vi "Controller - State Process.vi"(8 "error in (no error)":errorcluster, 11 "View Model":T1) -> (0 "error out":errorcluster, 3 "View Model":T1)   [LabVIEW 2017]
doc: "Process state during car wash execution."
uses:
  View Model/Controls/View Model.ctl
  View Model/Controls/Shared Model.ctl
  Error Handler/Controls/Error Model.ctl
  Error Handler/Controls/Error Data.ctl
  Error Handler/Controls/Error Level.ctl
  Configuration/Controls/Config Model.ctl
  Configuration/Controls/Config Record.ctl
  Configuration/Controls/Config Data.ctl
  Configuration/Controls/Config Command.ctl
  Controls/Controler Model.ctl
  Views/Entry Console View/Controls/Entry Console - Wash Steps.ctl
  Controls/Controller - Event.ctl
  Controls/Controller - Commands.ctl
  Controls/Controller - Overhead.ctl
  Controls/Controller - States.ctl
  Controls/Controller - Wash Step.ctl
  Views/Vehicle Position View/Controls/Vehicle - Station Enum.ctl
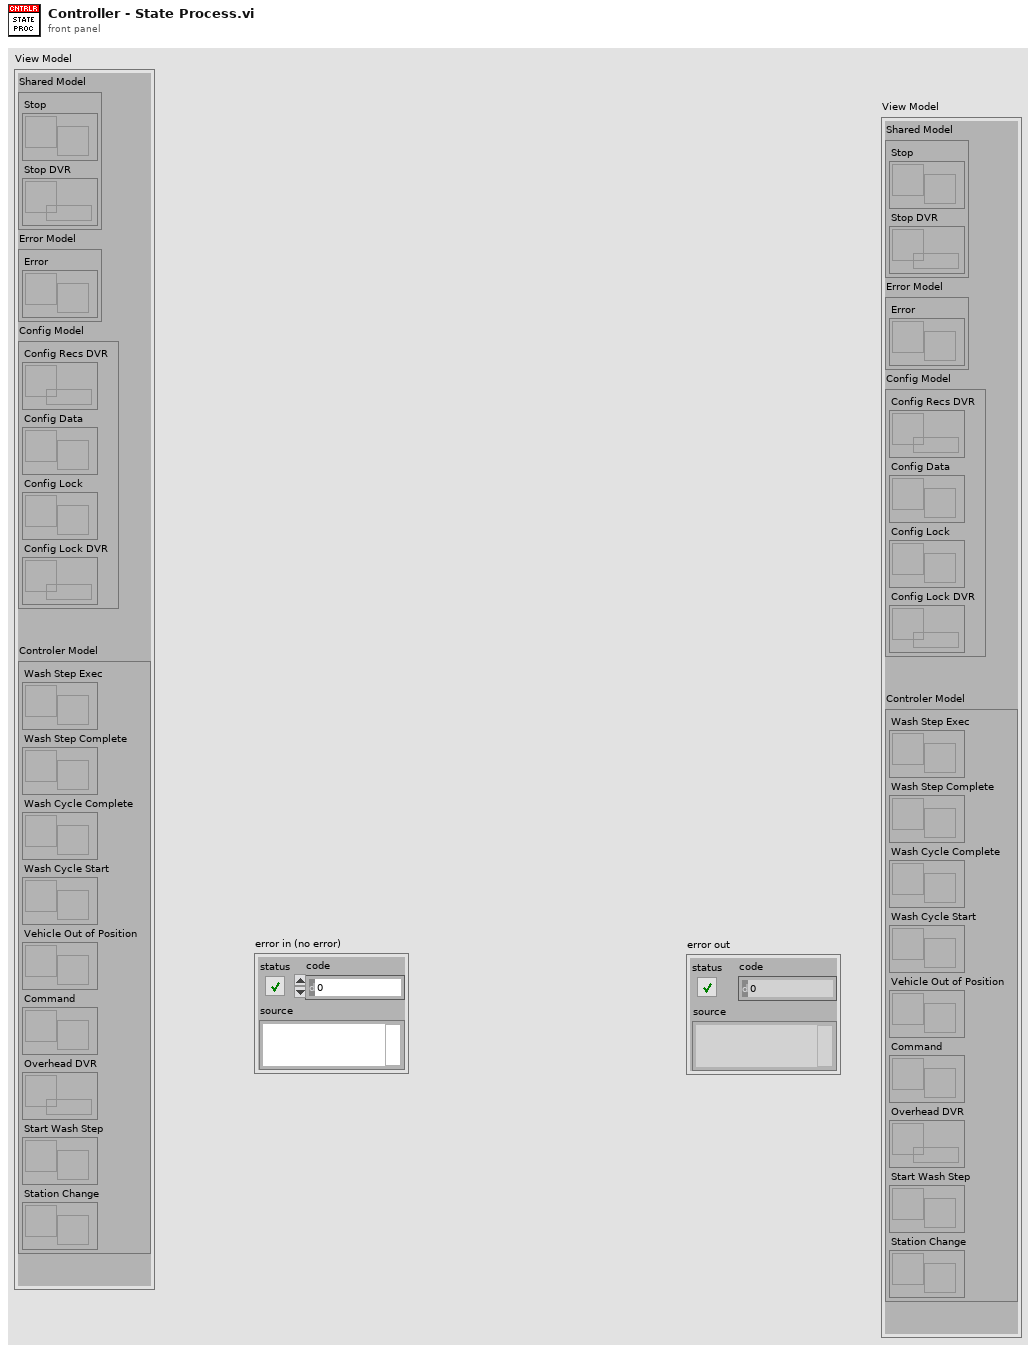
[diagram p1: front panel]
types:
  T1 = typedef "View Model.ctl" = cluster{"Shared Model":T2, "Error Model":T3, "Config Model":T4, "Controler Model":T5}
  T2 = typedef "Shared Model.ctl" = cluster{"Stop":refnum<user-event>, "Stop DVR":refnum<data-value>}
  T3 = typedef "Error Model.ctl" = cluster{"Error":refnum<user-event>}
  T4 = typedef "Config Model.ctl" = cluster{"Config Recs DVR":refnum<data-value>, "Config Data":refnum<user-event>, "Config Lock":refnum<user-event>, "Config Lock DVR":refnum<data-value>}
  T5 = typedef "Controler Model.ctl" = cluster{"Wash Step Exec":refnum<user-event>, "Wash Step Complete":refnum<user-event>, "Wash Cycle Complete":refnum<user-event>, "Wash Cycle Start":refnum<user-event>, "Vehicle Out of Position":refnum<user-event>, "Command":refnum<user-event>, "Overhead DVR":refnum<data-value>, "Start Wash Step":refnum<user-event>, "Station Change":refnum<user-event>}
  T6 = typedef "Controller - States.ctl" = enum16{"Initial", "Wait for Start", "Wash Cycle Start", "Wait for Vehicle Position", "Wash Step Start", "Wash Step Execute", "Wash Step Complete", "Wash Cycle Complete", "Wash Exit", "Wash Abort/Terminate"}
  T7 = typedef "Controller - Wash Step.ctl" = enum16{"Under Body Wash", "Bug Remover", "Pre-Soak", "High Pressure Wash", "Low Pressure Wax", "Spot Free Rinse", "Tire Shine Foam", "Air Dry"}
  T8 = typedef "Config Record.ctl" = cluster{"Wash Step":string, "Station":string, "Step Duration":u32}
  T9 = typedef "Vehicle - Station Enum.ctl" = enum16{"Entry", "Station1", "Station2", "Station3", "Exit"}
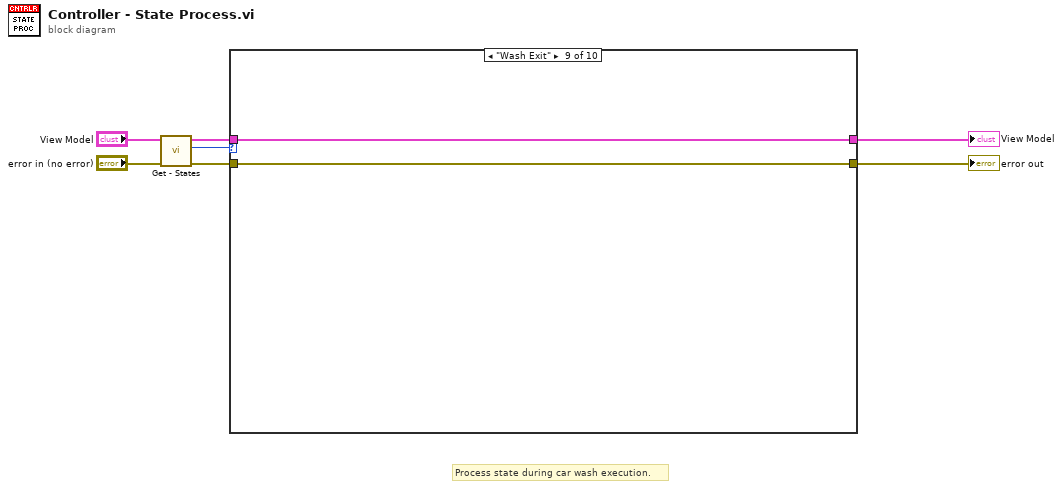
[diagram p0: block diagram]
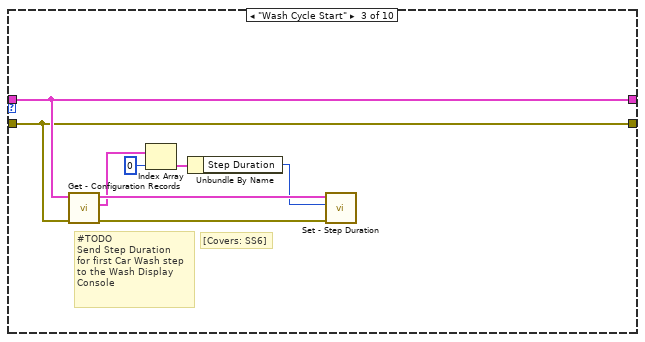
[diagram p4: hidden frame]
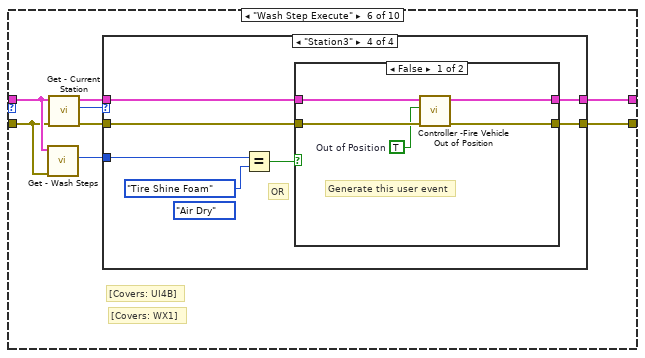
[diagram p7: hidden frame]
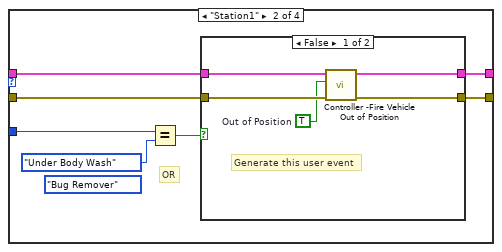
[diagram p9: hidden frame]
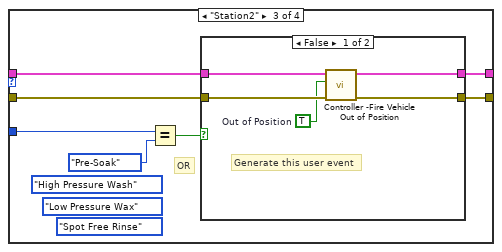
[diagram p11: hidden frame]
diagram:
  # "Process state during car wash execution."
  n1 = call "Get - States.vi"("error in (no error)"="error in (no error)", "View Model"="View Model") -> ("error out"=w3:errorcluster, "Current State"=w5:T6, "View Model"=w4:T1)  [unwired: 6 in, 1 out]
  n2 = case shown="\"Wash Exit\"" w5 {
    tunnel: w4 -> [w9 w11 w17 w21 w23 w28 w77 w79 w81 w83]
    tunnel: w3 -> [w8 w10 w16 w20 w22 w27 w76 w78 w80 w82]
    tunnel: [w9 w11 w17 w21 w23 w25 w77 w79 w81 w83] -> w1
    tunnel: [w8 w10 w16 w20 w22 w24 w76 w78 w80 w82] -> w2
    frame "Initial" {
    }
    frame "Wait for Start", Default {
      # "[Covers: WS1]"
      # "#TODO\n- Continue maintain Initial state requirements"
    }
    frame "Wash Cycle Start" {
      # "[Covers: SS6]"
      # "#TODO\nSend Step Duration\nfor first Car Wash step\nto the Wash Display \nConsole"
      n3 = call "Get - Configuration Records.vi"("error in (no error)"=w16, "View Model"=w17) -> ("error out"=w12:errorcluster, "Config Records"=w15:T8[], "View Model"=w18:T1)  [unwired: 7 in]
      n4 = Index Array(array=w15, index=0) -> (element=w14:T8)
      n5 = Unbundle By Name(w14) -> ("Step Duration"=w13:u32)
      n6 = call "Set - Step Duration.vi"("error in (no error)"=w12, "Step Duration"=w13, "View Model"=w18) -> ()  [unwired: 7 in, 2 out]
    }
    frame "Wait for Vehicle Position" {
      # "[Covers: VS4]"
      # "#TODO\nWait for user event Station\nChange to the correct station\nor to the Exit"
    }
    frame "Wash Step Start" {
    }
    frame "Wash Step Execute" {
      # "[Covers: WX1]"
      # "[Covers: UI4B]"
      n7 = call "Get - Wash Steps.vi"("error in (no error)"=w27, "View Model"=w28) -> ("Current Wash Step"=w26:T7)  [unwired: 6 in, 3 out]
      n8 = call "Get - Current Station.vi"("error in (no error)"=w27, "View Model"=w28) -> ("error out"=w30:errorcluster, "Current Station"=w31:T9, "View Model"=w29:T1)  [unwired: 7 in]
      n9 = case shown="\"Station3\"" w31 {
        tunnel: w30 -> [w32 w35 w49 w63]
        tunnel: w29 -> [w33 w37 w51 w65]
        tunnel: w26 -> [_ w40 w54 w68]
        tunnel: [w33 w36 w50 w64] -> w25
        tunnel: [w32 w34 w48 w62] -> w24
        frame "Entry", Default {
        }
        frame "Station1" {
          (unwired) Controller_-_Wash_Step."Bug Remover" ("Current Wash Step")
          # "OR"
          n10 = Equal?(x=w40, y=Controller_-_Wash_Step."Under Body Wash" ("Current Wash Step")) -> (x = y?=w38:bool)
          n11 = case shown="False" w38 {
            tunnel: w37 -> [w45 w47]
            tunnel: [w44 w47] -> w36
            tunnel: w35 -> [w43 w46]
            tunnel: [w42 w46] -> w34
            frame False {
              w41 = TRUE  # Out of Position
              # "Generate this user event"
              n12 = call "Controller -Fire Vehicle Out of Position.vi"("error in (no error)"=w43, "Out of Position"=w41, "View Model"=w45) -> ("error out"=w42:errorcluster, "View Model"=w44:T1)  [unwired: 7 in]
            }
            frame True {
              # "#TODO\nExecute current Car Wash Step"
            }
          }
        }
        frame "Station2" {
          (unwired) Controller_-_Wash_Step."Spot Free Rinse" ("Current Wash Step")
          (unwired) Controller_-_Wash_Step."Low Pressure Wax" ("Current Wash Step")
          (unwired) Controller_-_Wash_Step."High Pressure Wash" ("Current Wash Step")
          # "OR"
          n13 = Equal?(x=w54, y=Controller_-_Wash_Step."Pre-Soak" ("Current Wash Step")) -> (x = y?=w52:bool)
          n14 = case shown="False" w52 {
            tunnel: w51 -> [w59 w61]
            tunnel: [w58 w61] -> w50
            tunnel: w49 -> [w57 w60]
            tunnel: [w56 w60] -> w48
            frame False {
              w55 = TRUE  # Out of Position
              # "Generate this user event"
              n15 = call "Controller -Fire Vehicle Out of Position.vi"("error in (no error)"=w57, "Out of Position"=w55, "View Model"=w59) -> ("error out"=w56:errorcluster, "View Model"=w58:T1)  [unwired: 7 in]
            }
            frame True {
              # "#TODO\nExecute current Car Wash Step"
            }
          }
        }
        frame "Station3" {
          (unwired) Controller_-_Wash_Step."Air Dry" ("Current Wash Step")
          # "OR"
          n16 = Equal?(x=w68, y=Controller_-_Wash_Step."Tire Shine Foam" ("Current Wash Step")) -> (x = y?=w66:bool)
          n17 = case shown="False" w66 {
            tunnel: w65 -> [w73 w75]
            tunnel: [w72 w75] -> w64
            tunnel: w63 -> [w71 w74]
            tunnel: [w70 w74] -> w62
            frame False {
              w69 = TRUE  # Out of Position
              # "Generate this user event"
              n18 = call "Controller -Fire Vehicle Out of Position.vi"("error in (no error)"=w71, "Out of Position"=w69, "View Model"=w73) -> ("error out"=w70:errorcluster, "View Model"=w72:T1)  [unwired: 7 in]
            }
            frame True {
              # "#TODO\nExecute current Car Wash Step"
            }
          }
        }
      }
    }
    frame "Wash Step Complete" {
      # "[Covers: WC3C]"
      # "#TODO\nWait for user move the car to the correct station\nfor next wash step execution.\nStation Change event"
    }
    frame "Wash Cycle Complete" {
      # "[Covers: WC2C]"
      # "#TODO\nWait for user move the car to the Exit position\nStation Change event = Exit"
    }
    frame "Wash Exit" {
    }
    frame "Wash Abort/Terminate" {
    }
  }
  "error out" <- w2
  "View Model" <- w1
